vi "ErrorLatch.vi"(2 "Error Message":string, 3 "Trigger":bool) -> (1 "Latched":bool)   [LabVIEW 2020]
doc: "This VI will latch an error flag until cleared or suppressed (overriden). This VI is designed for integration with global variables to read the error clear and override signals."
uses:
  driverdata.vi
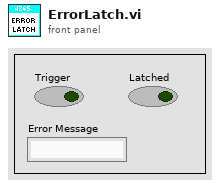
[diagram p1: front panel]
types:
  T1 = enum16{"Center", "North", "NorthWest", "West", "SouthWest", "South", "SouthEast", "East", "NorthEast"}
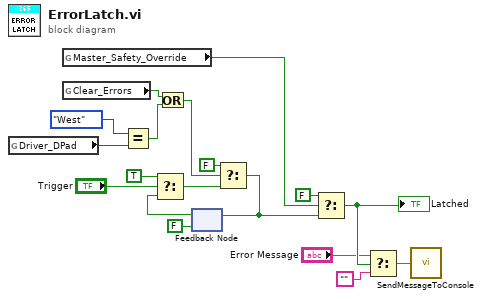
[diagram p0: block diagram]
diagram:
  n1 = global read "driverdata.vi" "Driver_DPad"() -> (w6:T1)
  n2 = global read "driverdata.vi" "Master_Safety_Override"() -> (w10:bool)
  n3 = global read "driverdata.vi" "Clear_Errors"() -> (w9:bool)
  n4 = Equal?(x=T1."West" ("Driver_DPad"), y=w6) -> (x = y?=w5:bool)
  n5 = Or(x=w9, y=w5) -> (x .or. y?=w8:bool)
  n6 = feedback #1(FALSE) -> (w17:bool)
  n7 = Select(t=TRUE, s="Trigger", f=w17) -> (s? t:f=w14:bool)
  n8 = Select(t=FALSE, s=w8, f=w14) -> (s? t:f=w12:bool)
  n9 = feedback-in #1(w12) -> ()
  n10 = Select(t=FALSE, s=w10, f=w12) -> (s? t:f=w4:bool)
  "Latched" <- w4
  n11 = Select(t="Error Message", s=w4, f="") -> (s? t:f=w2:string)
  n12 = call "SendMessageToConsole.vi"("Message String"=w2) -> ()  [unwired: 1 in]
